vi "ziExample-Module-MDS_DAQ.vi"() -> ()   [LabVIEW 2009]
doc: "This examples allows to control a Zurich Instruments device via a LabOne Labview API. \nThis vi enables the multi-device synchronisation of two ZI instruments of the same family.\n\n© Zurich Instruments AG, www.zhinst.com"
uses:
  <instrlib>/Zurich Instruments LabOne/Public/Modules/ziTypeModEnum.ctl
  <instrlib>/Zurich Instruments LabOne/Public/Modules/ziModSetValueDouble.vi
  <instrlib>/Zurich Instruments LabOne/Public/Modules/ziModSetValueDoubleArray.vi
  <instrlib>/Zurich Instruments LabOne/Public/Modules/ziModSetValueBinary.vi
  <instrlib>/Zurich Instruments LabOne/Public/Modules/ziModGetDoubleData.vi
  <instrlib>/Zurich Instruments LabOne/Public/Utility/ziTicksToS_vector.vi
  <instrlib>/Zurich Instruments LabOne/Zurich Instruments LabOne.lvlib
panel:
  in  "subscribe":string[](array[string])=["demods/0/sample.R", "demods/0/sample.AuxIn1"] caption="Subscribe Paths"
  out "DoubleSample":T1
  in  "stop":bool
  out "XY Graph":cluster{"Timestamp(s)":dbl[], "Value":dbl[]}[](graph)
  in  "noofpoints":i32=10 caption="Number of Points"
  in  "duration":dbl=1.0 caption="Duration (s)"
  out "Error Out":errorcluster
  in  "Follower":string[](array[string])=["dev"]
  out "Status":dbl
  out "Message":string
  in  "Leader":string="dev"
  # "ziExample-Module-MDS_DAQ.vi\nRequirements: 2x(MFLI or UHF or HDAWG )\nsee block diagram for VI description"
  # "Tested Devices:\n\n- MFLI\n- UHF"
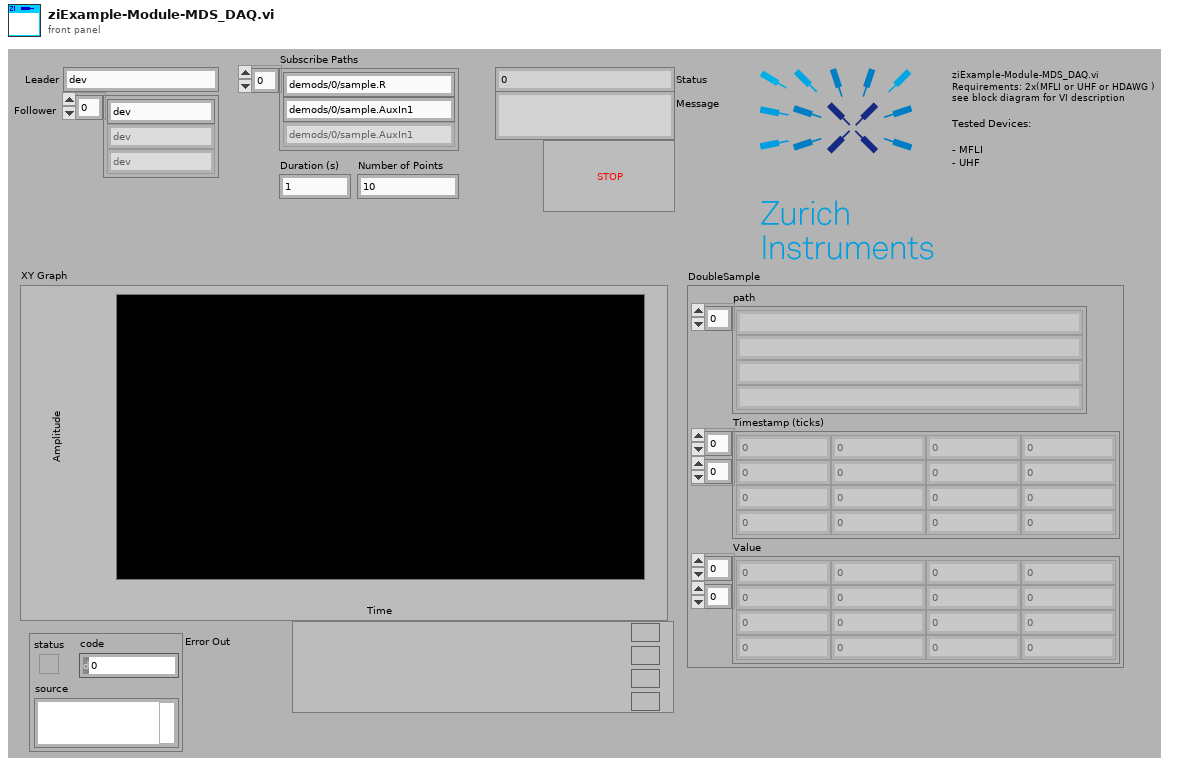
[diagram p1: front panel]
types:
  T1 = cluster{"path":string[], "Timestamp (ticks)":u64[][], "Value":dbl[][]}
  T2 = typedef "Zurich Instruments LabOne.lvlib/ziTypeModEnum.ctl" = u16
  T3 = typedef "Zurich Instruments LabOne.lvlib/ziTypeHandle.ctl" = cluster{"handleValid":bool, "Conn":u64, "Path Prefix":string, "Handle":u64, "Connected":bool, "Clockbase(s)":dbl}
  T4 = typedef "Zurich Instruments LabOne.lvlib/ziTypeModHandle.ctl" = cluster{"handleValid":bool, "Conn":u64, "ModHandle":u64, "moduleID":string, "Path Prefix":string}
  T5 = typedef "Zurich Instruments LabOne.lvlib/ziTypeModResults.ctl" = cluster{"PathArray":string[], "ValueType":T6, "NoOfResults":u64, "ziGenericHeader":T7[]}
  T6 = typedef "Zurich Instruments LabOne.lvlib/ziTypePollType.ctl" = enum16{"NONE", "DOUBLE_DATA", "INTEGER_DATA", "DEMOD_SAMPLE", "SCOPE_WAVE_HF2", "AUXIN_SAMPLE", "DIO_SAMPLE", "BYTE_ARRAY", "PWA_WAVE", "9", "10", "11", "12", "13", "14", "15", "TREE_CHANGE_DEPRI", "17", "ERROR", "19", "20", "21", "22", "23", "24", "25", "26", "27", "28", "29", "30", "31", "DOUBLE_DATA_TS", "INTEGER_DATA_TS", "34", "SCOPE_WAVE", "SCOPE_WAVE_EX", "37", "BYTE_ARRAY_TS", "39", "40", "41", "42", "43", "44", "45", "CNT_DATA", "47", "TREE_CHANGE", "49", "50", "51", "52", "53", "54", "55", "56", "57", "58", "59", "60", "61", "62", "63", "SWEEPER_DATA", "SPECTRUM_DATA", "ADVISOR_DATA", "VECTOR_DATA", "IMP_DATA"}
  T7 = typedef "Zurich Instruments LabOne.lvlib/ziTypeModGenericHeader.ctl" = cluster{"HeaderType":enum8{"HEADER_TYPE_NONE", "HEADER_TYPE_SWTRIGGER", "HEADER_TYPE_SWEEPER"}, "SampleFormat":u8, "SystemTime":timestamp, "CreatedTimeStamp":u64, "ChangedTimeStamp":u64, "Flags":u32, "ChunkSizeBytes":u64, "Name":string, "Status":u32, "GroupIndex":u32, "Color":u32, "ActiveRow":u32, "TriggerNumber":u64, "GridRows":u32, "GridCols":u32, "GridMode":u32, "GridOperation":u32, "GridDirection":u32, "GridRepetitions":u32, "GridColDelta":dbl, "GridColOffset":dbl, "GridRowDelta":dbl, "GridRowOffset":dbl, "Bandwidth":dbl, "Center":dbl, "Nenbw":dbl}
  T8 = typedef "Zurich Instruments LabOne.lvlib/ziTypeDoubleDataTS.ctl" = cluster{"Timestamp (ticks)":u64[], "Value":dbl[]}
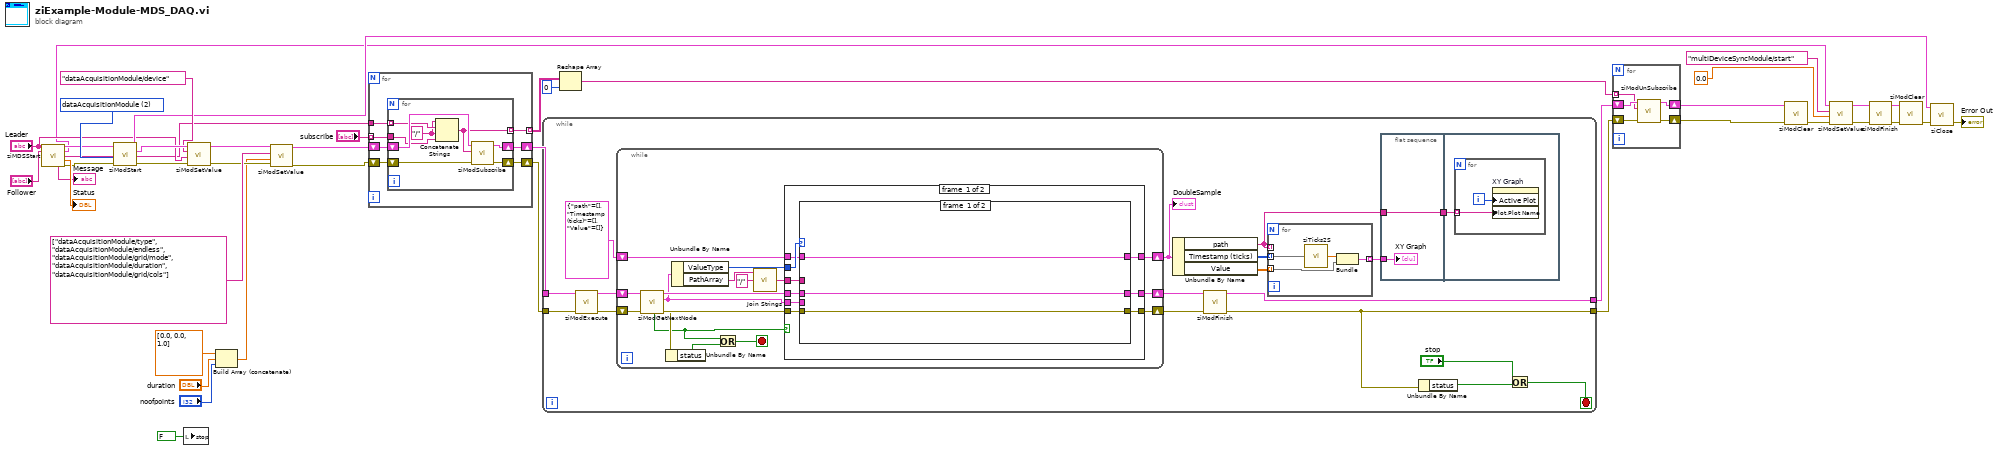
[diagram p0: block diagram]
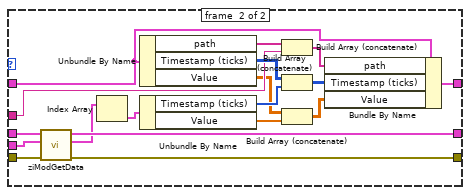
[diagram p2: hidden frame]
diagram:
  w20 = T2 2 items=["sweep", "scopeModule", "dataAcquisitionModule", "pidAdvisor", "awgModule", "impedanceModule", "multiDeviceSyncModule", "zoomFFT", "trigger", "deviceSettings", "record"] ("module Id")
  n1 = call <instrlib>:"ziMDSStart.vi"("Master"="Leader", "Slaves"="Follower") -> ("Handle Out"=w14:T3, "ModHandle Out"=w6:T4, "MDS_Devices"=w10:string[], "Status"=→"Status":dbl, "Message"=→"Message":string, "Error Out"=w13:errorcluster)  [unwired: 8 in]
  n2 = call <instrlib>:"ziModStart.vi"("Error In"=w13, "module Id"=w20, "Handle In"=w14) -> ("Error Out"=w34:errorcluster, "ModHandle Out"=w35:T4, "Handle Out"=w16:T3)  [unwired: 6 in]
  n3 = local write "stop"(FALSE ("run")) -> ()
  n4 = call-poly <instrlib>:"ziModSetValue.vi"("Error In"=w34, "Data"="Leader", "Path"="dataAcquisitionModule/device", "ModHandle In"=w35) -> ("Error Out"=w29:errorcluster, "ModHandle Out"=w30:T4)  [unwired: 6 in]
  n5 = Build Array (concatenate)(dbl[] [0.0, 0.0, 1.0], "duration", "noofpoints") -> (w21:dbl[])
  n6 = call-poly <instrlib>:"ziModSetValue.vi"("Error In"=w29, "Values"=w21, "Paths"=string[] ["dataAcquisitionModule/type", "dataAcquisitionModule/endless", "dataAcquisitionModule/grid/mode", "dataAcquisitionModule/duration", "dataAcquisitionModule/grid/cols"], "ModHandle In"=w30) -> ("Error Out"=w25:errorcluster, "ModHandle Out"=w26:T4)  [unwired: 6 in]
  n7 = for {
    tunnel: "subscribe" -> [w45] mode=indexing
    shift-right: [w49] -> w28
    shift-left: w26 -> [w47]
    shift-right: [w48] -> w27
    shift-left: w25 -> [w46]
    tunnel: w10 -> [w44]
    tunnel: [w43] -> w9 mode=indexing
    n8 = for {
      tunnel: w45 -> [w51]
      tunnel: w44 -> [w53] mode=indexing
      shift-right: [w56] -> w48
      shift-left: w46 -> [w54]
      shift-right: [w57] -> w49
      shift-left: w47 -> [w55]
      tunnel: [w50] -> w43 mode=indexing
      w52 = "/" ("string")
      n9 = Concatenate Strings(w52, w53, w52, w51) -> (w50:string)
      n10 = call <instrlib>:"ziModSubscribe.vi"("Error In"=w54, "Path"=w50, "ModHandle In"=w55) -> ("Error Out"=w56:errorcluster, "ModHandle Out"=w57:T4)  [unwired: 6 in]
    }
  }
  n11 = while {
    tunnel: [w61] -> w33
    tunnel: [w73] -> w32
    tunnel: w28 -> [w72]
    tunnel: w27 -> [w71]
    stop <- w58 stop-if-true
    n12 = call <instrlib>:"ziModExecute.vi"("Error In"=w71, "ziModHandle In"=w72) -> ("Error Out"=w69:errorcluster, "ziModHandle Out"=w70:T4)  [unwired: 6 in, 1 out]
    n13 = while {
      shift-right: [w96] -> w74
      shift-left: w70 -> [w100]
      shift-right: [w97] -> w75
      shift-left: w69 -> [w88]
      shift-right: [w90] -> w68
      shift-left: T1 {"path"=[], "Timestamp (ticks)"=[], "Value"=[]} ("DoubleSample") -> [w91]
      stop <- w85 stop-if-true
      n14 = call <instrlib>:"ziModGetNextNode.vi"("Error In"=w88, "ModHandle In"=w100) -> ("Error Out"=w98:errorcluster, "ModResults"=w95:T5, "ModHandle Out"=w99:T4, "NoData"=w87:bool)  [unwired: 6 in]
      n15 = Unbundle By Name(w88) -> ("status"=w86:bool)
      n16 = Unbundle By Name(w95) -> ("ValueType"=w92:T6, "PathArray"=w89:string[])
      n17 = Or(x=w87, y=w86) -> (x .or. y?=w85:bool)
      n18 = call <vilib>:"Join Strings.vi"("Separator (,)"="/", "Strings In"=w89) -> ("String"=w93:string)  [unwired: 1 in]
      n19 = case shown="False" w87 {
        tunnel: w95 -> [w109 _]
        tunnel: w99 -> [w108 w133]
        tunnel: w98 -> [w107 w132]
        tunnel: [w106 w132] -> w97
        tunnel: [w105 w133] -> w96
        tunnel: w93 -> [w101 _]
        tunnel: w92 -> [w104 _]
        tunnel: w91 -> [w103 w131]
        tunnel: [w102 w131] -> w90
        frame #0 {
          n20 = case shown="\"DOUBLE_DATA_TS\"" w104 {
            tunnel: w108 -> [w112 w127]
            tunnel: w109 -> [_ w126]
            tunnel: w107 -> [w111 w128]
            tunnel: [w111 w129] -> w106
            tunnel: [w112 w130] -> w105
            tunnel: w103 -> [w110 w116]
            tunnel: [w110 w117] -> w102
            tunnel: w101 -> [_ w119]
            frame #0 {
            }
            frame #1 {
              n21 = call-poly <instrlib>:"ziModGetData.vi"("Error In"=w128, "ModResults"=w126, "ModHandle In"=w127) -> ("Error Out"=w129:errorcluster, "DoubleSample"=w125:T8[], "ModHandle Out"=w130:T4)  [unwired: 4 in, 2 out]
              n22 = Index Array(array=w125) -> (element=w124:T8)  [unwired: 1 in]
              n23 = Unbundle By Name(w116) -> ("path"=w120:string[], "Timestamp (ticks)"=w123:u64[][], "Value"=w115:dbl[][])
              n24 = Unbundle By Name(w124) -> ("Timestamp (ticks)"=w122:u64[], "Value"=w114:dbl[])
              n25 = Build Array (concatenate)(w120, w119) -> (w118:string[])
              n26 = Build Array (concatenate)(w123, w122) -> (w121:u64[][])
              n27 = Build Array (concatenate)(w115, w114) -> (w113:dbl[][])
              n28 = Bundle By Name(cluster=w116, "path"=w118, "Timestamp (ticks)"=w121, "Value"=w113) -> (w117:T1)
            }
          }
        }
        frame #1 {
        }
      }
    }
    "DoubleSample" <- w68
    n29 = Unbundle By Name(w68) -> ("path"=w63:string[], "Timestamp (ticks)"=w67:u64[][], "Value"=w66:dbl[][])
    n30 = call <instrlib>:"ziModFinish.vi"("Error In"=w75, "ziModHandle In"=w74) -> ("Error Out"=w61:errorcluster, "ziModHandle Out"=w73:T4)  [unwired: 7 in]
    n31 = for {
      tunnel: w67 -> [w82] mode=indexing
      tunnel: w66 -> [w84] mode=indexing
      tunnel: [w83] -> w65 mode=indexing
      tunnel: w63 -> [_] mode=indexing
      n32 = call-poly <instrlib>:"ziTicks2S.vi"("Timestamp (ticks)"=w82) -> ("Timestamp(s)"=w81:dbl[])  [unwired: 2 in, 2 out]
      n33 = Bundle("Timestamp(s)"=w81, "Value"=w84) -> (w83:cluster{"Timestamp(s)":dbl[], "Value":dbl[]})  [unwired: 1 in]
    }
    n34 = flat-sequence {
      tunnel: w65 -> [w77]
      tunnel: [w76] -> w64
      tunnel: w63 -> [w76]
      tunnel: w64 -> [w78]
      frame #0 {
        "XY Graph" <- w77
      }
      frame #1 {
        n35 = for {
          tunnel: w78 -> [w80] mode=indexing
          i -> [w79]
          n36 = property on="XY Graph" class="XYGraph (strict)"("Active Plot"=w79, "Plot.Plot Name"=w80) -> ()  [unwired: 2 in, 2 out]
        }
      }
    }
    n37 = Unbundle By Name(w61) -> ("status"=w60:bool)
    n38 = Or(x="stop", y=w60) -> (x .or. y?=w58:bool)
  }
  n39 = Reshape Array(w9, 0 ("dimension size")) -> (w8:string[])
  n40 = for {
    tunnel: w8 -> [w134] mode=indexing
    shift-right: [w137] -> w37
    shift-left: w32 -> [w135]
    shift-right: [w138] -> w38
    shift-left: w33 -> [w136]
    n41 = call <instrlib>:"ziModUnSubscribe.vi"("Error In"=w136, "Path (\"/\")"=w134, "ModHandle In"=w135) -> ("Error Out"=w138:errorcluster, "ModHandle Out"=w137:T4)  [unwired: 7 in]
  }
  n42 = call <instrlib>:"ziModClear.vi"("Error In"=w38, "ziModHandle In"=w37) -> ("Error Out"=w3:errorcluster)  [unwired: 7 in, 1 out]
  n43 = call-poly <instrlib>:"ziModSetValue.vi"("Error In"=w3, "Value"=0.0, "Path"="multiDeviceSyncModule/start", "ModHandle In"=w6) -> ("Error Out"=w2:errorcluster, "ModHandle Out"=w5:T4)  [unwired: 6 in]
  n44 = call <instrlib>:"ziModFinish.vi"("Error In"=w2, "ziModHandle In"=w5) -> ("Error Out"=w42:errorcluster, "ziModHandle Out"=w41:T4)  [unwired: 7 in]
  n45 = call <instrlib>:"ziModClear.vi"("Error In"=w42, "ziModHandle In"=w41) -> ("Error Out"=w12:errorcluster)  [unwired: 7 in, 1 out]
  n46 = call <instrlib>:"ziClose.vi"("Error In"=w12, "Handle In"=w16) -> ("Error Out"=→"Error Out":errorcluster)  [unwired: 2 in, 1 out]
